vi "One-Shot Boolean Toggle Switch.vi"(1 "Toggle Button Input":bool) -> (0 "New Toggled Output":bool)   [LabVIEW 2019]
uses:
  Toggle Switch Variable.vi
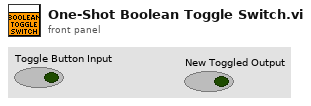
[diagram p1: front panel]
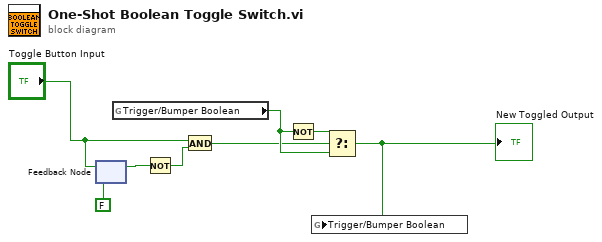
[diagram p0: block diagram]
diagram:
  n1 = feedback #1(FALSE) -> (w2:bool)
  n2 = feedback-in #1("Toggle Button Input") -> ()
  n3 = global read "Toggle Switch Variable.vi" "Trigger/Bumper Boolean"() -> (w6:bool)
  n4 = Not(x=w2) -> (.not. x?=w1:bool)
  n5 = And(x="Toggle Button Input", y=w1) -> (x .and. y?=w5:bool)
  n6 = Not(x=w6) -> (.not. x?=w7:bool)
  n7 = Select(t=w7, s=w5, f=w6) -> (s? t:f=w8:bool)
  "New Toggled Output" <- w8
  n8 = global write "Toggle Switch Variable.vi" "Trigger/Bumper Boolean"(w8) -> ()
